vi "Get Failure set to write.vi"(11 "Failure set":string[](array[string])) -> (3 "Failure set to write":string)   [LabVIEW 2023]
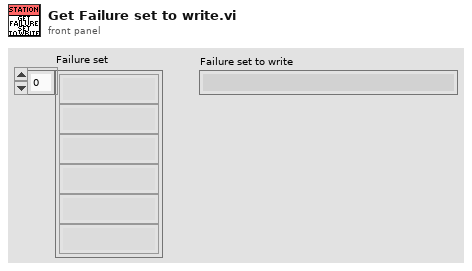
[diagram p1: front panel]
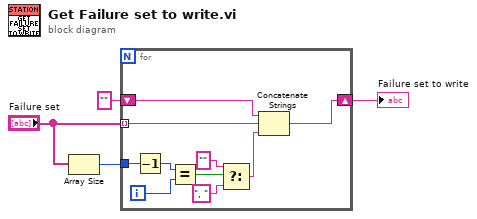
[diagram p0: block diagram]
diagram:
  n1 = Array Size(array="Failure set") -> (size(s)=w3:i32)
  n2 = for {
    tunnel: "Failure set" -> [w14] mode=indexing
    tunnel: w3 -> [w13]
    shift-right: [w5] -> w1
    shift-left: "" -> [w6]
    i -> [w11]
    n3 = Decrement(x=w13) -> (x-1=w12:i32)
    n4 = Equal?(x=w12, y=w11) -> (x = y?=w10:bool)
    n5 = Select(t="", s=w10, f=", ") -> (s? t:f=w9:string)
    n6 = Concatenate Strings(w6, w14, w9) -> (w5:string)
  }
  "Failure set to write" <- w1
